vi "Get Broadcasts.vi"(8 "error in (no error)":errorcluster, 11 "Timeout (10 sec)":u32=10) -> (0 "error out":errorcluster, 2 "Timeout?":bool, 3 "GMOD Broadcast List":T1)   [LabVIEW 2015, in "Generic Module Library.lvlib" / "Template G_Module.lvlib"]
uses:
  Template G_Module.lvlib
  Private API/Module Broadcasts/Broadcast Support/Broadcast Actions.ctl
  Private Controls/Event Item.ctl
  Private API/Module Broadcasts/API/Broadcast List.ctl
panel:
  # "DO NOT MANUALLY CHANGE THIS NAME"
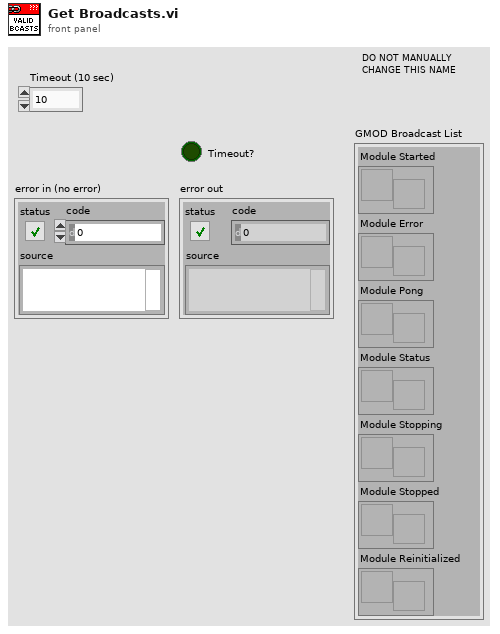
[diagram p1: front panel]
types:
  T1 = typedef "Generic Module Library.lvlib/Template G_Module.lvlib/Broadcast List.ctl" = cluster{"Module Started":refnum<user-event>, "Module Error":refnum<user-event>, "Module Pong":refnum<user-event>, "Module Status":refnum<user-event>, "Module Stopping":refnum<user-event>, "Module Stopped":refnum<user-event>, "Module Reinitialized":refnum<user-event>}
  T2 = typedef "Generic Module Library.lvlib/Template G_Module.lvlib/Broadcast Actions.ctl" = enum16{"Create", "Get", "Destroy"}
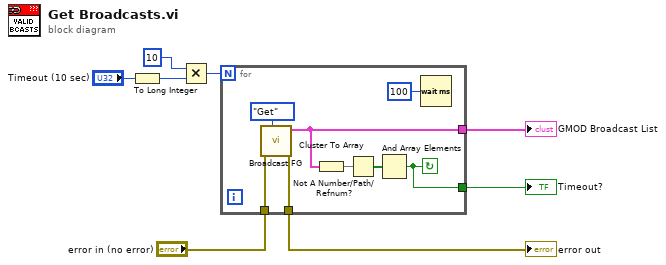
[diagram p0: block diagram]
diagram:
  n1 = To Long Integer(number="Timeout (10 sec)") -> (32bit integer=w6:i32)
  n2 = Multiply(x=10, y=w6) -> (x*y=w5:i32)
  n3 = for {
    N: w5 -> [_]
    tunnel: "error in (no error)" -> [w14]
    tunnel: [w13] -> w1
    tunnel: [w11] -> w3
    tunnel: [w9] -> w2
    stop <- w11 continue-if-true
    n4 = call "Broadcast FG.vi"("Broadcast Actions"=Broadcast_Actions."Get", "error in"=w14) -> ("error out"=w13:errorcluster, "Broadcast List"=w9:T1)  [unwired: 8 in]
    n5 = Cluster To Array(cluster=w9) -> (array=w10:refnum<user-event>[])
    n6 = Not A Number/Path/Refnum?(number/path/refnum=w10) -> (NaN/Path/Refnum?=w15:bool[])
    n7 = And Array Elements(Boolean array=w15) -> (logical AND=w11:bool)
    n8 = Wait (ms)(milliseconds to wait=u32 100) -> ()  [unwired: 1 out]
  }
  "error out" <- w1
  "Timeout?" <- w3
  "GMOD Broadcast List" <- w2
